vi "OP6_SCARICO.vi"(0 "Esito 2 in":cluster{"Si":bool, "No":bool}, 1 "Esito 3 in":cluster{"Si":bool, "No":bool}, 2 "Esito 4 in":cluster{"Si":bool, "No":bool}, 3 "Esito 5 in":cluster{"Si":bool, "No":bool}, 4 "Esito 6 in":cluster{"Si":bool, "No":bool}, 5 "Esito 7 in":cluster{"Si":bool, "No":bool}, 6 "Esito 8 in":cluster{"Si":bool, "No":bool}, 7 "Esito 9 in":cluster{"Si":bool, "No":bool}, 8 "Esito 1 in":cluster{"Si":bool, "No":bool}, 9 "Tasto premuto":T1(array[ring]), 10 "Tipo specifica":string, 12 "Stato in":u16, 14 "Stato out":u16) -> (15 "scrivi":bool, 16 "Dato":string[](array[string]), 17 "ANNULLA PROVA":bool, 18 "Esito 1 out":T2, 19 "i out":i32=1, 20 "Esito 2 out":T2, 21 "Esito 3 out":T2, 22 "Esito 4 out":T2, 23 "Esito 5 out":T2, 24 "Esito 6 out":T2, 25 "Esito 7 out":T2, 26 "Esito 8 out":T2, 27 "Esito 9 out":T2)   [LabVIEW 2022 SP3]
uses:
  Labview/Globali.vi
panel:
  in  "i max":i32
  in  "i":i32=1
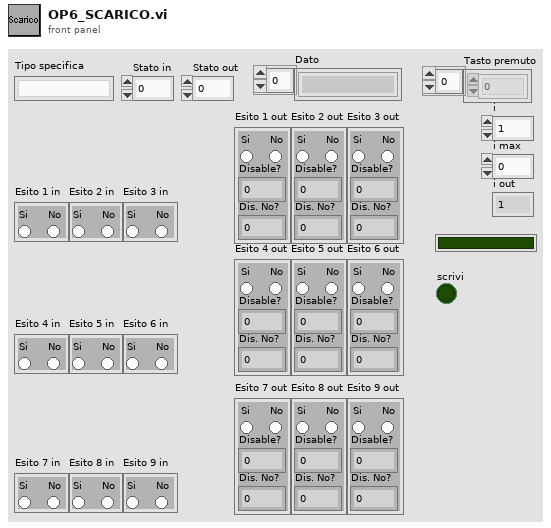
[diagram p1: front panel]
types:
  T1 = enum16{"0", "1", "2", "3", "4", "5", "6", "7", "8", "9", "A", "B", "C", "D", "E", "F", "G", "H", "I", "J", "K", "L", "M", "N", "O", "P", "Q", "R", "S", "T", "U", "V", "W", "X", "Y", "Z", "F1", "F2", "F3", "F4", "F5", "F6", "F7", "F8", "F9", "F10", "F11", "F12", "F13", "F14", "F15", "ADD", "BACK", "BACKSLASH", "CAPITAL", "COMMA", "DECIMAL", "DELETE", "DIVIDE", "DOWN", "END", "EQUALS", "ESCAPE", "GRAVE (`)", "HOME", "INSERT", "LBRACKET", "LCONTROL", "LEFT", "L ALT", "LSHIFT", "LWIN", "MINUS", "MULTIPLY", "NEXT", "NUMLOCK", "NUMPAD_0", "NUMPAD_1", "NUMPAD_2", "NUMPAD_3", "NUMPAD_4", "NUMPAD_5", "NUMPAD_6", "NUMPAD_7", "NUMPAD_8", "NUMPAD_9", "PAUSE", "PERIOD", "PRIOR (PG UP)", "RBRACKET", "RCONTROL", "RETURN", "RIGHT", "R ALT", "RSHIFT", "RWIN", "SCROLL", "SEMICOLON", "SLASH", "SPACE", "SUBTRACT", "TAB", "UP", "ENTER (num pad)", "' (quote)"}[]
  T2 = cluster{"Disable?":i16, "Si":bool, "No":bool, "Dis. No?":i16}
  T3 = cluster{"Esito 1 out":cluster{"Disable?":i16, "Si":bool, "No":bool, "Dis. No?":i16}, "Esito 2 out":cluster{"Disable?":i16, "Si":bool, "No":bool, "Dis. No?":i16}, "Esito 3 out":cluster{"Disable?":i16, "Si":bool, "No":bool, "Dis. No?":i16}, "Esito 4 out":cluster{"Disable?":i16, "Si":bool, "No":bool, "Dis. No?":i16}, "Esito 5 out":cluster{"Disable?":i16, "Si":bool, "No":bool, "Dis. No?":i16}, "Esito 6 out":cluster{"Disable?":i16, "Si":bool, "No":bool, "Dis. No?":i16}, "Esito 7 out":cluster{"Disable?":i16, "Si":bool, "No":bool, "Dis. No?":i16}, "Esito 8 out":cluster{"Disable?":i16, "Si":bool, "No":bool, "Dis. No?":i16}, "Esito 9 out":cluster{"Disable?":i16, "Si":bool, "No":bool, "Dis. No?":i16}}
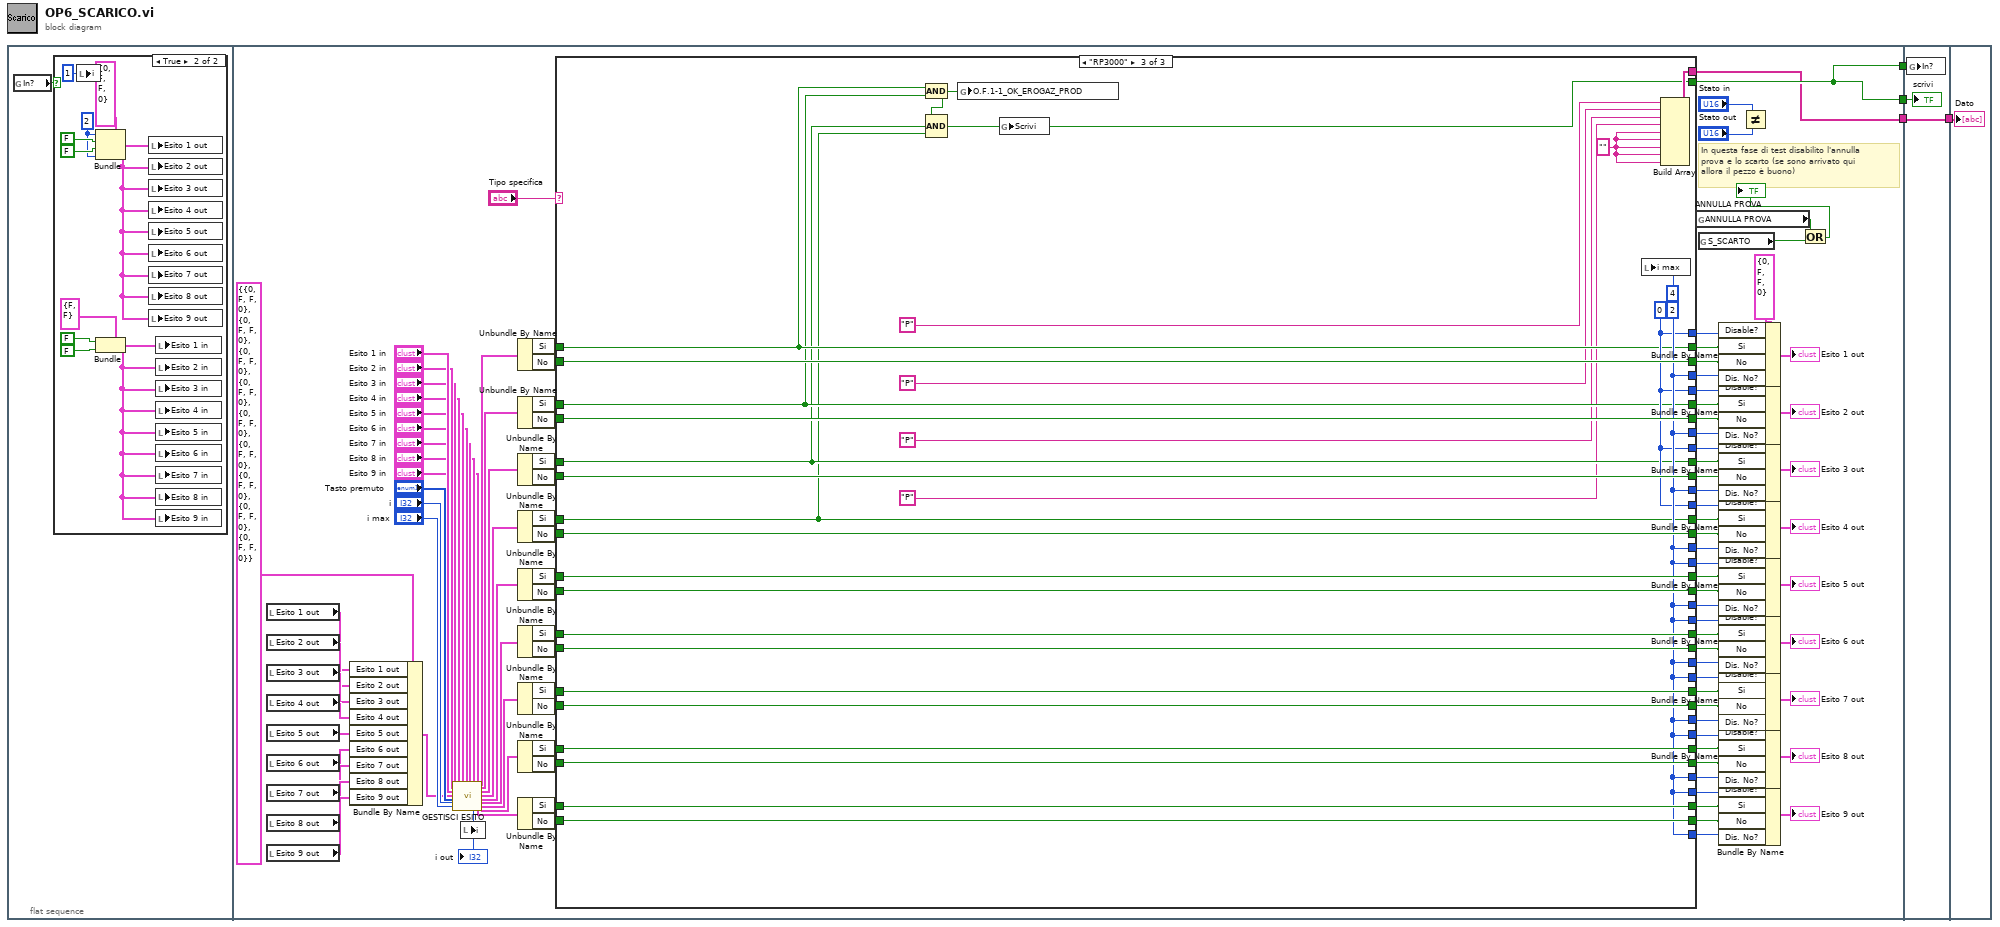
[diagram p0: block diagram]
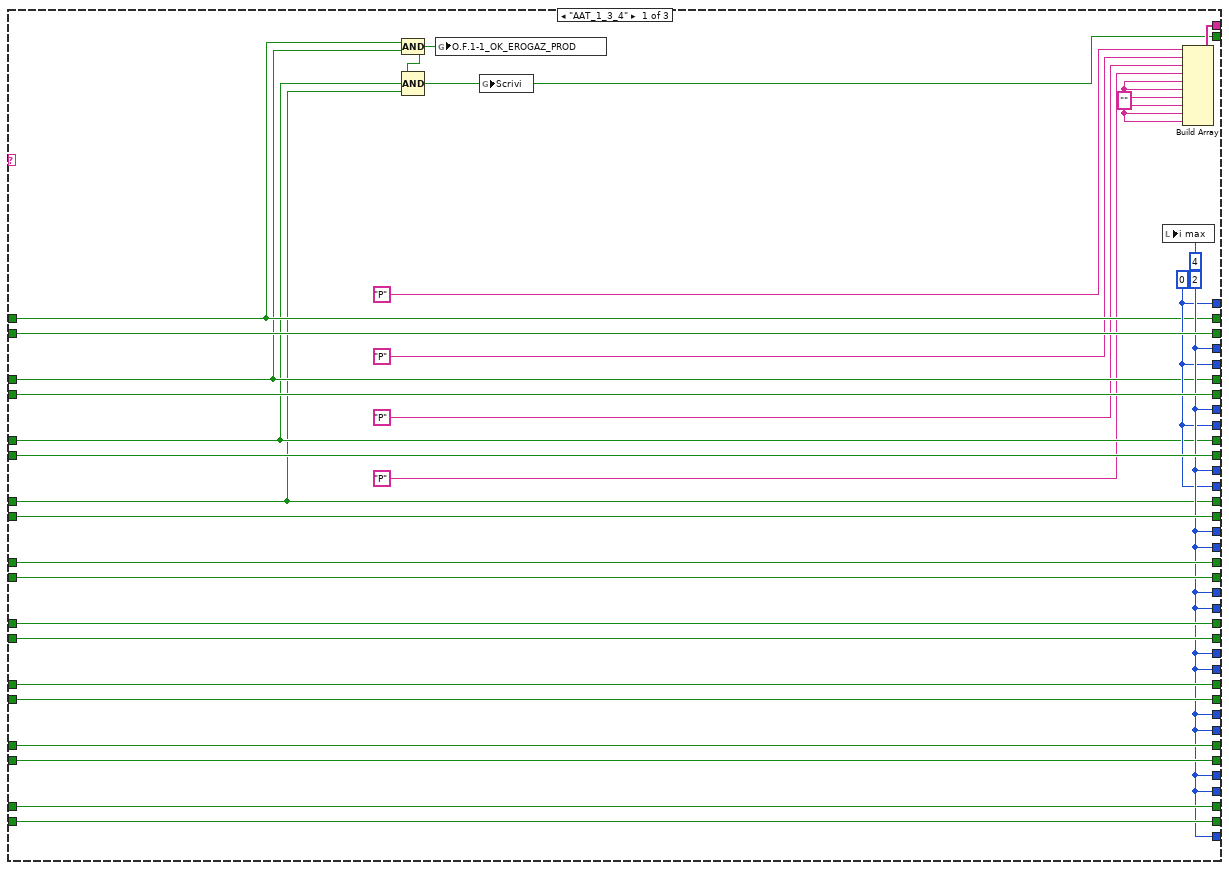
[diagram p3: hidden frame]
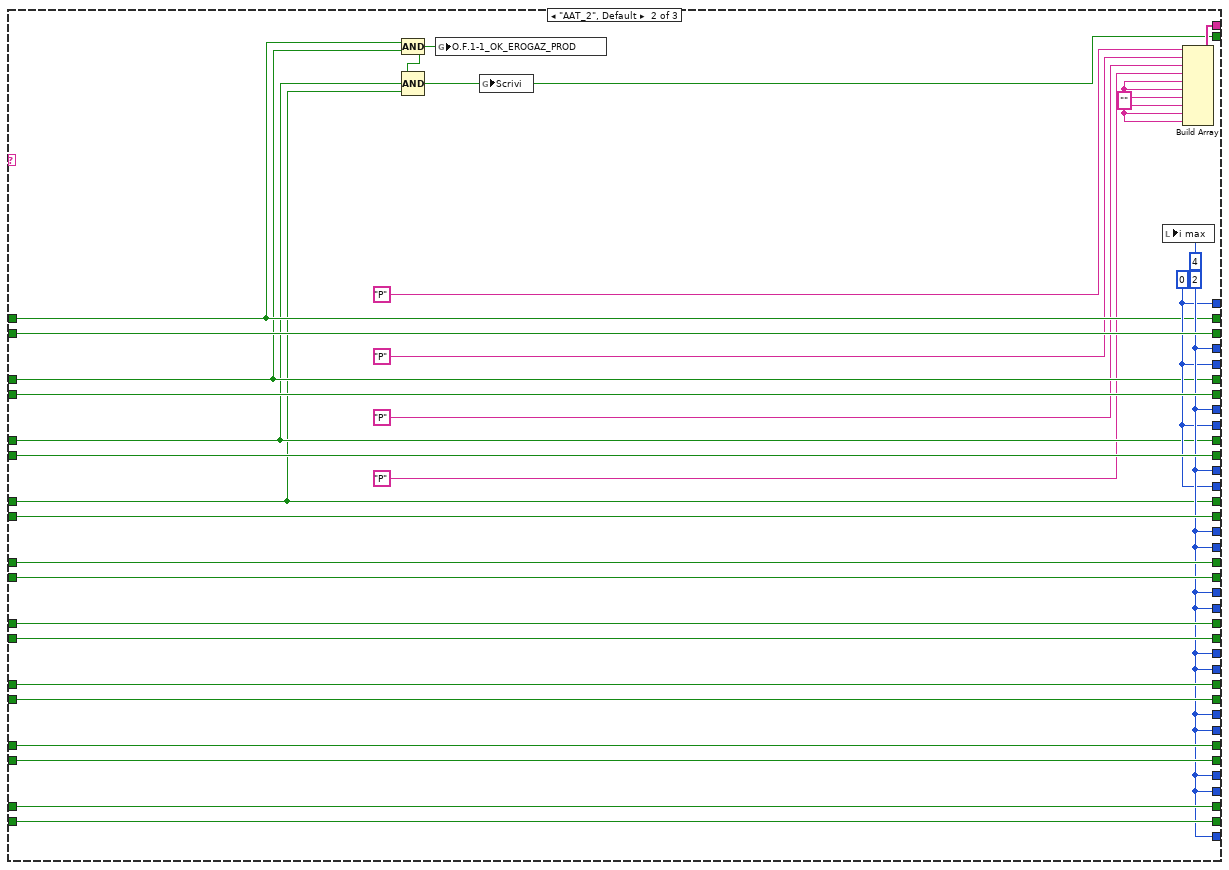
[diagram p4: hidden frame]
diagram:
  n1 = flat-sequence {
    tunnel: [w17] -> w4
    tunnel: [w17] -> w3
    tunnel: [w16] -> w1
    tunnel: w4 -> [w210]
    tunnel: w3 -> [w209]
    tunnel: [w208] -> w2
    tunnel: w1 -> [w208]
    tunnel: w2 -> [w211]
    frame #0 {
      n2 = global read "Globali.vi" "In?"() -> (w5:bool)
      n3 = case shown="True" w5 {
        frame False {
        }
        frame True {
          w12 = i16 2 ("Disable?")
          n4 = local write "i"(1 ("i")) -> ()
          n5 = Bundle(cluster=T2 {"Disable?"=0, "Si"=FALSE, "No"=FALSE, "Dis. No?"=0} ("Esito 1 out"), "Disable?"=w12, "Si"=FALSE, "No"=FALSE, "Dis. No?"=w12) -> (w11:T2)
          n6 = Bundle(cluster=cluster{"Si":bool, "No":bool} {"Si"=FALSE, "No"=FALSE} ("Esito 1 in"), "Si"=FALSE, "No"=FALSE) -> (w9:cluster{"Si":bool, "No":bool})
          n7 = local write "Esito 1 out"(w11) -> ()
          n8 = local write "Esito 2 out"(w11) -> ()
          n9 = local write "Esito 3 out"(w11) -> ()
          n10 = local write "Esito 4 out"(w11) -> ()
          n11 = local write "Esito 5 out"(w11) -> ()
          n12 = local write "Esito 6 out"(w11) -> ()
          n13 = local write "Esito 7 out"(w11) -> ()
          n14 = local write "Esito 8 out"(w11) -> ()
          n15 = local write "Esito 9 out"(w11) -> ()
          n16 = local write "Esito 1 in"(w9) -> ()
          n17 = local write "Esito 2 in"(w9) -> ()
          n18 = local write "Esito 3 in"(w9) -> ()
          n19 = local write "Esito 4 in"(w9) -> ()
          n20 = local write "Esito 5 in"(w9) -> ()
          n21 = local write "Esito 6 in"(w9) -> ()
          n22 = local write "Esito 7 in"(w9) -> ()
          n23 = local write "Esito 8 in"(w9) -> ()
          n24 = local write "Esito 9 in"(w9) -> ()
        }
      }
    }
    frame #1 {
      w63 = T2 {"Disable?"=0, "Si"=FALSE, "No"=FALSE, "Dis. No?"=0} ("Esito 1 out")
      # "In questa fase di test disabilito l'annulla \nprova e lo scarto (se sono arrivato qui \nallora il pezzo è buono)"
      n25 = local read "Esito 1 out"() -> (w41:T2)
      n26 = local read "Esito 2 out"() -> (w42:T2)
      n27 = local read "Esito 3 out"() -> (w43:T2)
      n28 = local read "Esito 4 out"() -> (w44:T2)
      n29 = local read "Esito 5 out"() -> (w45:T2)
      n30 = local read "Esito 6 out"() -> (w46:T2)
      n31 = local read "Esito 7 out"() -> (w47:T2)
      n32 = local read "Esito 8 out"() -> (w48:T2)
      n33 = local read "Esito 9 out"() -> (w49:T2)
      n34 = Bundle By Name(cluster=T3 {"Esito 1 out"={"Disable?"=0, "Si"=FALSE, "No"=FALSE, "Dis. No?"=0}, "Esito 2 out"={"Disable?"=0, "Si"=FALSE, "No"=FALSE, "Dis. No?"=0}, "Esito 3 out"={"Disable?"=0, "Si"=FALSE, "No"=FALSE, "Dis. No?"=0}, "Esito 4 out"={"Disable?"=0, "Si"=FALSE, "No"=FALSE, "Dis. No?"=0}, "Esito 5 out"={"Disable?"=0, "Si"=FALSE, "No"=FALSE, "Dis. No?"=0}, "Esito 6 out"={"Disable?"=0, "Si"=FALSE, "No"=FALSE, "Dis. No?"=0}, "Esito 7 out"={"Disable?"=0, "Si"=FALSE, "No"=FALSE, "Dis. No?"=0}, "Esito 8 out"={"Disable?"=0, "Si"=FALSE, "No"=FALSE, "Dis. No?"=0}, "Esito 9 out"={"Disable?"=0, "Si"=FALSE, "No"=FALSE, "Dis. No?"=0}} ("Cluster"), "Esito 1 out"=w41, "Esito 2 out"=w42, "Esito 3 out"=w43, "Esito 4 out"=w44, "Esito 5 out"=w45, "Esito 6 out"=w46, "Esito 7 out"=w47, "Esito 8 out"=w48, "Esito 9 out"=w49) -> (w50:T3)
      n35 = call "GESTISCI ESITO.vi"("Esito 3 in"="Esito 3 in", "Esito 2 in"="Esito 2 in", "Esito 1 in"="Esito 1 in", "Cluster"=w50, "Tasto premuto"="Tasto premuto", "i in"="i", "i max"="i max", "Esito 4 in"="Esito 4 in", "Esito 5 in"="Esito 5 in", "Esito 6 in"="Esito 6 in", "Esito 7 in"="Esito 7 in", "Esito 8 in"="Esito 8 in", "Esito 9 in"="Esito 9 in") -> ("i out"=w21:i32, "Esito 9 in 2"=w39:cluster{"Si":bool, "No":bool}, "Esito 1 in 2"=w31:cluster{"Si":bool, "No":bool}, "Esito 2 in 2"=w32:cluster{"Si":bool, "No":bool}, "Esito 3 in 2"=w33:cluster{"Si":bool, "No":bool}, "Esito 4 in 2"=w34:cluster{"Si":bool, "No":bool}, "Esito 5 in 2"=w35:cluster{"Si":bool, "No":bool}, "Esito 6 in 2"=w36:cluster{"Si":bool, "No":bool}, "Esito 7 in 2"=w37:cluster{"Si":bool, "No":bool}, "Esito 8 in 2"=w38:cluster{"Si":bool, "No":bool})  [unwired: 5 in]
      "i out" <- w21
      n36 = local write "i"(w21) -> ()
      n37 = Unbundle By Name(w31) -> ("Si"=w84:bool, "No"=w83:bool)
      n38 = Unbundle By Name(w32) -> ("Si"=w67:bool, "No"=w68:bool)
      n39 = Unbundle By Name(w33) -> ("Si"=w69:bool, "No"=w70:bool)
      n40 = Unbundle By Name(w34) -> ("Si"=w71:bool, "No"=w72:bool)
      n41 = Unbundle By Name(w35) -> ("Si"=w73:bool, "No"=w74:bool)
      n42 = Unbundle By Name(w36) -> ("Si"=w75:bool, "No"=w76:bool)
      n43 = Unbundle By Name(w37) -> ("Si"=w77:bool, "No"=w78:bool)
      n44 = Unbundle By Name(w38) -> ("Si"=w79:bool, "No"=w80:bool)
      n45 = Unbundle By Name(w39) -> ("Si"=w81:bool, "No"=w82:bool)
      n46 = case shown="\"RP3000\"" "Tipo specifica" {
        tunnel: [w128 w157 w193] -> w16
        tunnel: [w134 w163 w190] -> w111
        tunnel: [w134 w163 w190] -> w110
        tunnel: [w134 w163 w190] -> w109
        tunnel: [w134 w163 w190] -> w108
        tunnel: [w135 w164 w192] -> w107
        tunnel: [w135 w164 w192] -> w106
        tunnel: [w135 w164 w192] -> w105
        tunnel: [w135 w164 w192] -> w104
        tunnel: [w135 w164 w192] -> w103
        tunnel: [w132 w161 w189] -> w102
        tunnel: [w139 w168 w197] -> w101
        tunnel: [w131 w160 w188] -> w100
        tunnel: [w140 w169 w198] -> w99
        tunnel: [w130 w159 w187] -> w98
        tunnel: [w149 w178 w207] -> w97
        tunnel: [w129 w158 w186] -> w96
        tunnel: [w148 w177 w206] -> w95
        tunnel: [w138 w167 w196] -> w94
        tunnel: [w147 w176 w205] -> w93
        tunnel: [w137 w166 w195] -> w92
        tunnel: [w146 w175 w204] -> w91
        tunnel: [w136 w165 w194] -> w90
        tunnel: [w145 w174 w203] -> w89
        tunnel: [w144 w173 w202] -> w88
        tunnel: [w143 w172 w201] -> w87
        tunnel: [w142 w171 w200] -> w86
        tunnel: [w141 w170 w199] -> w85
        tunnel: w84 -> [w132 w161 w189]
        tunnel: w83 -> [w139 w168 w197]
        tunnel: w82 -> [w141 w170 w199]
        tunnel: w81 -> [w142 w171 w200]
        tunnel: w80 -> [w143 w172 w201]
        tunnel: w79 -> [w144 w173 w202]
        tunnel: w78 -> [w145 w174 w203]
        tunnel: w77 -> [w136 w165 w194]
        tunnel: w76 -> [w146 w175 w204]
        tunnel: w75 -> [w137 w166 w195]
        tunnel: w74 -> [w147 w176 w205]
        tunnel: w73 -> [w138 w167 w196]
        tunnel: w72 -> [w148 w177 w206]
        tunnel: w71 -> [w129 w158 w186]
        tunnel: w70 -> [w149 w178 w207]
        tunnel: w69 -> [w130 w159 w187]
        tunnel: w68 -> [w140 w169 w198]
        tunnel: w67 -> [w131 w160 w188]
        tunnel: [w135 w164 w192] -> w62
        tunnel: [w135 w164 w192] -> w61
        tunnel: [w135 w164 w192] -> w60
        tunnel: [w135 w164 w192] -> w59
        tunnel: [w135 w164 w192] -> w58
        tunnel: [w135 w164 w192] -> w57
        tunnel: [w135 w164 w192] -> w56
        tunnel: [w135 w164 w192] -> w55
        tunnel: [w135 w164 w192] -> w54
        tunnel: [w125 w154 w183] -> w17
        frame "AAT_1_3_4" {
          w127 = ""
          w135 = 2
          w134 = 0
          n47 = Compound Arithmetic op=AND(w132, w131) -> (w133:bool)
          n48 = Compound Arithmetic op=AND(w133, w130, w129) -> (w125:bool)
          n49 = global write "Globali.vi" "O.F.1-1_OK_EROGAZ_PROD"(w133) -> ()
          n50 = global write "Globali.vi" "Scrivi"(w125) -> ()
          n51 = local write "i max"(4) -> ()
          n52 = Build Array("P", "P", "P", "P", w127, w127, w127, w127, w127, w127) -> (w128:string[])
        }
        frame "AAT_2", Default {
          w156 = ""
          w164 = 2
          w163 = 0
          n53 = Compound Arithmetic op=AND(w161, w160) -> (w162:bool)
          n54 = Compound Arithmetic op=AND(w162, w159, w158) -> (w154:bool)
          n55 = global write "Globali.vi" "O.F.1-1_OK_EROGAZ_PROD"(w162) -> ()
          n56 = global write "Globali.vi" "Scrivi"(w154) -> ()
          n57 = local write "i max"(4) -> ()
          n58 = Build Array("P", "P", "P", "P", w156, w156, w156, w156, w156, w156) -> (w157:string[])
        }
        frame "RP3000" {
          w191 = ""
          w192 = 2
          w190 = 0
          n59 = Compound Arithmetic op=AND(w189, w188) -> (w185:bool)
          n60 = Compound Arithmetic op=AND(w185, w187, w186) -> (w183:bool)
          n61 = global write "Globali.vi" "O.F.1-1_OK_EROGAZ_PROD"(w185) -> ()
          n62 = global write "Globali.vi" "Scrivi"(w183) -> ()
          n63 = local write "i max"(4) -> ()
          n64 = Build Array("P", "P", "P", "P", w191, w191, w191, w191, w191) -> (w193:string[])
        }
      }
      n65 = global read "Globali.vi" "ANNULLA PROVA"() -> (w19:bool)
      n66 = global read "Globali.vi" "S_SCARTO"() -> (w20:bool)
      n67 = Bundle By Name(cluster=w63, "Disable?"=w111, "Si"=w102, "No"=w101, "Dis. No?"=w62) -> (→"Esito 1 out":T2)
      n68 = Bundle By Name(cluster=w63, "Disable?"=w110, "Si"=w100, "No"=w99, "Dis. No?"=w61) -> (→"Esito 2 out":T2)
      n69 = Bundle By Name(cluster=w63, "Disable?"=w109, "Si"=w98, "No"=w97, "Dis. No?"=w60) -> (→"Esito 3 out":T2)
      n70 = Bundle By Name(cluster=w63, "Disable?"=w108, "Si"=w96, "No"=w95, "Dis. No?"=w59) -> (→"Esito 4 out":T2)
      n71 = Bundle By Name(cluster=w63, "Disable?"=w107, "Si"=w94, "No"=w93, "Dis. No?"=w58) -> (→"Esito 5 out":T2)
      n72 = Bundle By Name(cluster=w63, "Disable?"=w106, "Si"=w92, "No"=w91, "Dis. No?"=w57) -> (→"Esito 6 out":T2)
      n73 = Bundle By Name(cluster=w63, "Disable?"=w105, "Si"=w90, "No"=w89, "Dis. No?"=w56) -> (→"Esito 7 out":T2)
      n74 = Bundle By Name(cluster=w63, "Disable?"=w104, "Si"=w88, "No"=w87, "Dis. No?"=w55) -> (→"Esito 8 out":T2)
      n75 = Bundle By Name(cluster=w63, "Disable?"=w103, "Si"=w86, "No"=w85, "Dis. No?"=w54) -> (→"Esito 9 out":T2)
      n76 = Not Equal?(x="Stato in", y="Stato out") -> ()  [unwired: 1 out]
      n77 = Or(x=w19, y=w20) -> (x .or. y?=→"ANNULLA PROVA":bool)
    }
    frame #2 {
      n78 = global write "Globali.vi" "In?"(w210) -> ()
      "scrivi" <- w209
    }
    frame #3 {
      "Dato" <- w211
    }
  }
